vi "ElevFF_MinAchieveVelocity.vi"(9 "Acceleration":dbl, 10 "MaxVoltage":dbl, 11 "in ELEV_FF":T1 {"Kg" format="%13.5p"; "Ka" format="%13.5p"; "Kv" format="%13.5p"; "Ks" format="%13.5p"}) -> (3 "MinVelocity":dbl)   [LabVIEW 2019, in "Trajectory_Library.lvlib"]
doc: "Calculates the minimum achievable velocity given a maximum voltage supply and an acceleration. Useful for ensuring that velocity and acceleration constraints for a trapezoidal profile are simultaneously achievable - enter the acceleration constraint, and this will give you a simultaneously-achievable velocity constraint.\n \nInputs: \n - ElevFF -- The ElevFF data cluster\n - maxVoltage -- The maximum voltage that can be supplied to the elevator.\n - acceleration -- The acceleration of the elevator.\n\nOutputs:\n - MinVelocity -- The minimum possible velocity at the given acceleration."
uses:
  Trajectory_Library.lvlib
  TypeDef/ELEV_FF.ctl
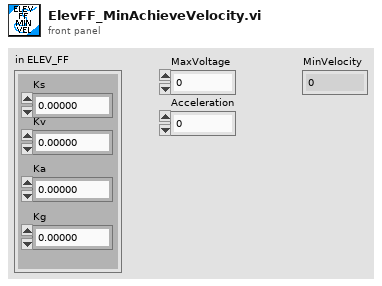
[diagram p1: front panel]
types:
  T1 = typedef "Trajectory_Library.lvlib/ELEV_FF.ctl" = cluster{"Ks":dbl, "Kv":dbl, "Ka":dbl, "Kg":dbl}
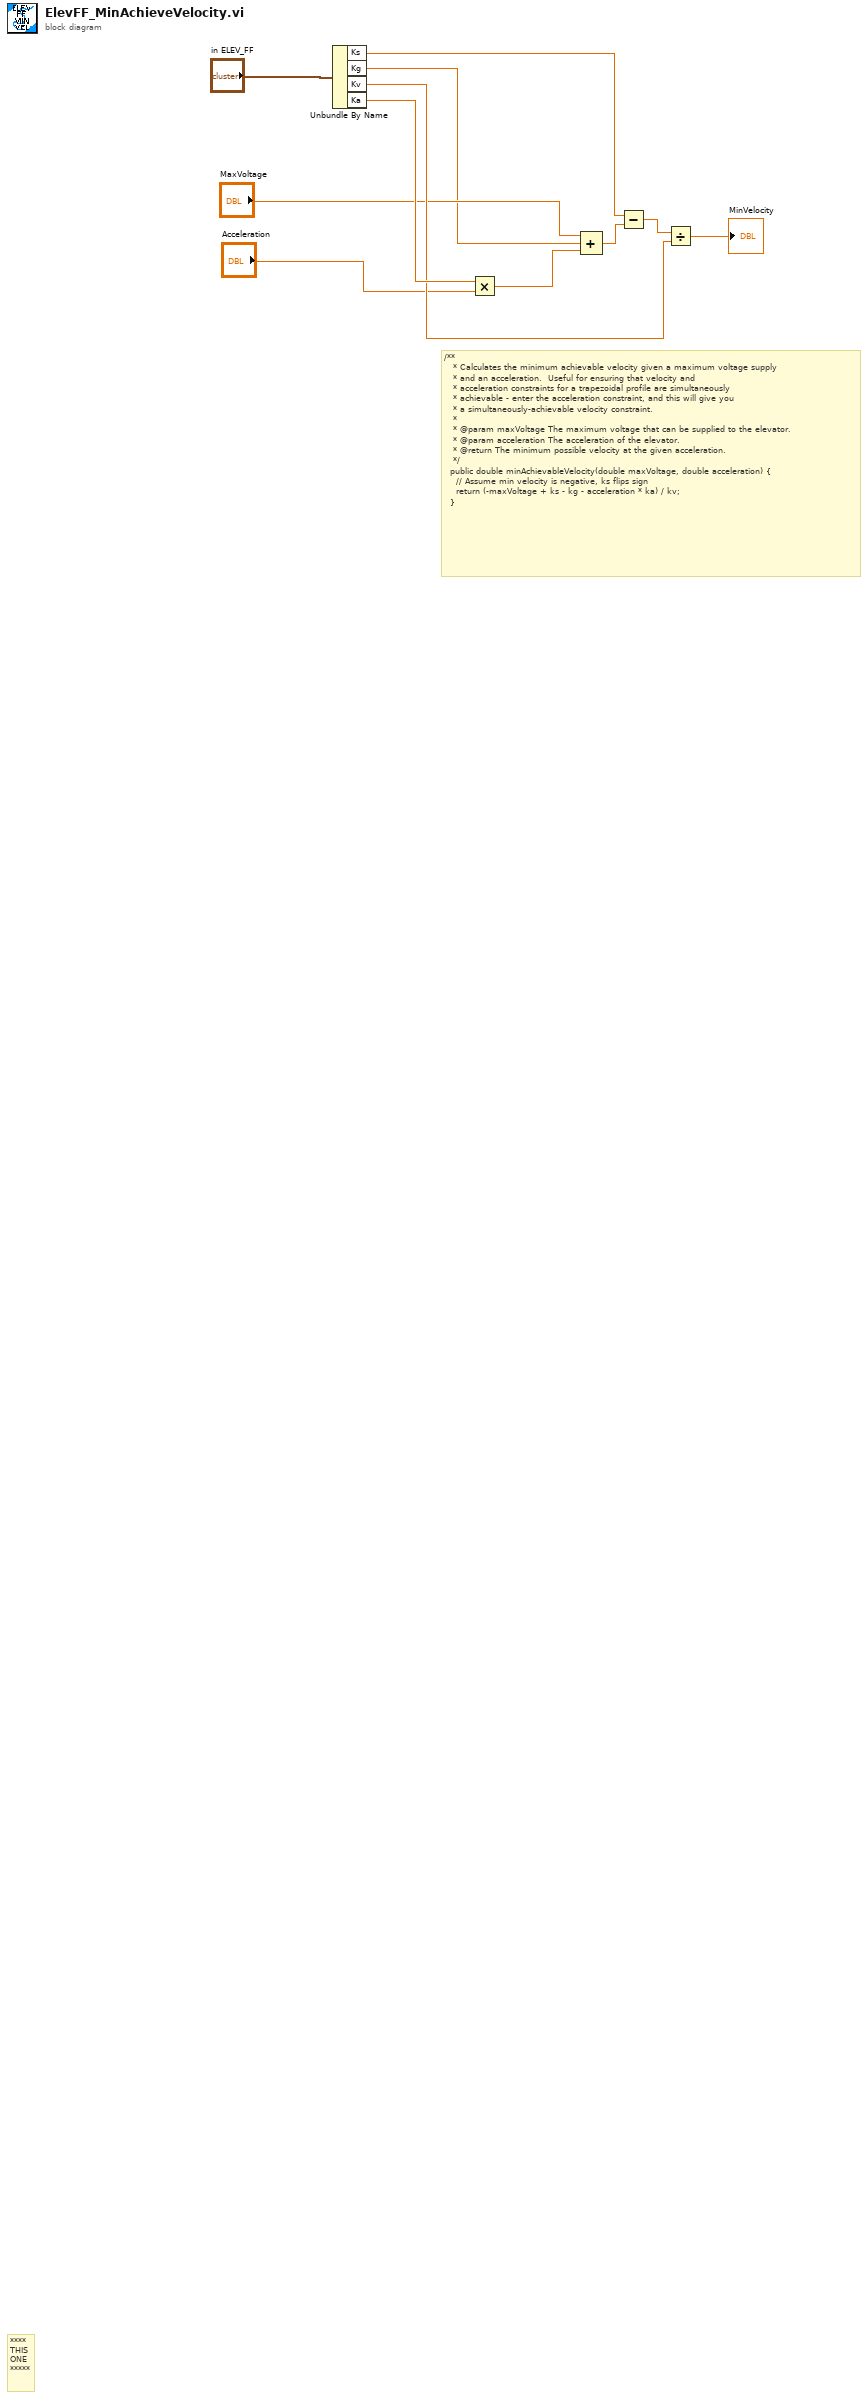
[diagram p0: block diagram]
diagram:
  # "/**\n   * Calculates the minimum achievable velocity given a maximum voltage supply\n   * and an acceleration.  Useful for ensuring that velocity and\n   * acceleration constraints for a trapezoidal profile are simultaneously\n   * achievable - enter the acceleration constraint, and this will give you\n   * a simultaneously-achievable velocity constraint.\n   *\n   * @param maxVoltage The maximum voltage that can be supplied to the elevator.\n   * @param acceleration The acceleration of the elevator.\n   * @return The minimum possible velocity at the given acceleration.\n   */\n  public double minAchievableVelocity(double maxVoltage, double acceleration) {\n    // Assume min velocity is negative, ks flips sign\n    return (-maxVoltage + ks - kg - acceleration * ka) / kv;\n  }"
  # "****\nTHIS\nONE\n*****"
  n1 = Unbundle By Name("in ELEV_FF") -> ("Ks"=w5:dbl, "Kg"=w2:dbl, "Kv"=w7:dbl, "Ka"=w9:dbl)
  n2 = Multiply(x=w9, y="Acceleration") -> (x*y=w10:dbl)
  n3 = Compound Arithmetic op=ADD("MaxVoltage", w2, w10) -> (w4:dbl)
  n4 = Subtract(x=w5, y=w4) -> (x-y=w6:dbl)
  n5 = Divide(x=w6, y=w7) -> (x/y=→"MinVelocity":dbl)
